vi "nav refnum registry.vi"(10 "Action":enum16{"Open", "Retreive", "Close"}(ring), 11 "nav type":i32) -> (1 "valid refnum?":bool, 3 "VI reference":refnum<vi>)   [LabVIEW 2009]
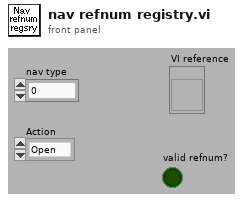
[diagram p1: front panel]
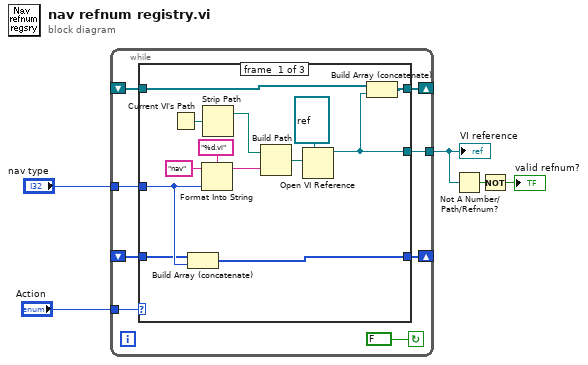
[diagram p0: block diagram]
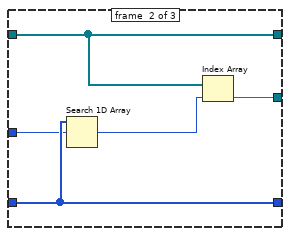
[diagram p2: hidden frame]
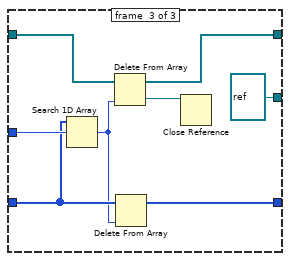
[diagram p3: hidden frame]
diagram:
  n1 = while {
    tunnel: "nav type" -> [w13]
    tunnel: [w12] -> w3
    tunnel: "Action" -> [w11]
    shift-right: [w10] -> _
    shift-left: _ -> [w9]
    shift-right: [w8] -> _
    shift-left: _ -> [w7]
    stop <- FALSE continue-if-true
    n2 = case shown="\"Close\"" w11 {
      tunnel: w13 -> [w17 w28 w38]
      tunnel: [w20 w30 refnum<vi> refnum ("type specifier VI Refnum (for type only)")] -> w12
      tunnel: [w19 w31 w35] -> w10
      tunnel: w9 -> [w18 w31 w39]
      tunnel: [w16 w29 w36] -> w8
      tunnel: w7 -> [w15 w29 w37]
      frame #0 {
        n3 = Current VI's Path() -> (path=w23:path)
        n4 = Build Array (concatenate)(w15, w17) -> (w16:i32[])
        n5 = Format Into String(format string="%d.vi", initial string="nav", w17) -> (resulting string=w24:string)  [unwired: 1 in, 1 out]
        n6 = Strip Path(path=w23) -> (stripped path=w22:path)  [unwired: 1 out]
        n7 = Build Path(base path=w22, name or relative path=w24) -> (appended path=w21:path)
        n8 = Open VI Reference(type specifier VI Refnum (for type only)=refnum<vi> refnum, vi path=w21) -> (vi reference=w20:refnum<vi>)  [unwired: 4 in, 1 out]
        n9 = Build Array (concatenate)(w18, w20) -> (w19:refnum<vi>[])
      }
      frame #1 {
        n10 = Search 1D Array(1D array=w29, element=w28) -> (index of element=w27:i32)  [unwired: 1 in]
        n11 = Index Array(array=w31, index=w27) -> (element=w30:refnum<vi>)
      }
      frame #2 {
        n12 = Search 1D Array(1D array=w37, element=w38) -> (index of element=w33:i32)  [unwired: 1 in]
        n13 = Delete From Array(array=w39, index=w33) -> (deleted portion=w34:refnum<vi>, array with subset deleted=w35:refnum<vi>[])  [unwired: 1 in]
        n14 = Delete From Array(array=w37, index=w33) -> (array with subset deleted=w36:i32[])  [unwired: 1 in, 1 out]
        n15 = Close Reference(reference=w34) -> ()  [unwired: 1 in, 1 out]
      }
    }
  }
  "VI reference" <- w3
  n16 = Not A Number/Path/Refnum?(number/path/refnum=w3) -> (NaN/Path/Refnum?=w4:bool)
  n17 = Not(x=w4) -> (.not. x?=→"valid refnum?":bool)
